vi "Global 1.vi"() -> ()   [LabVIEW 2015]
panel:
  in  "Received  Data":string
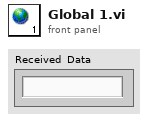
[diagram p1: front panel]
diagram:
